vi "Varint Decoder uint64.vi"(7 "Optional":bool, 8 "error in (no error)":errorcluster, 9 "Array":u8[](array[numeric]) format="%02x", 10 "Key":i32=-1) -> (0 "error out":errorcluster, 1 "array w/ subset deleted":u8[](array[numeric]), 2 "Read Key":i32, 3 "Varint":u64)   [LabVIEW 2017]
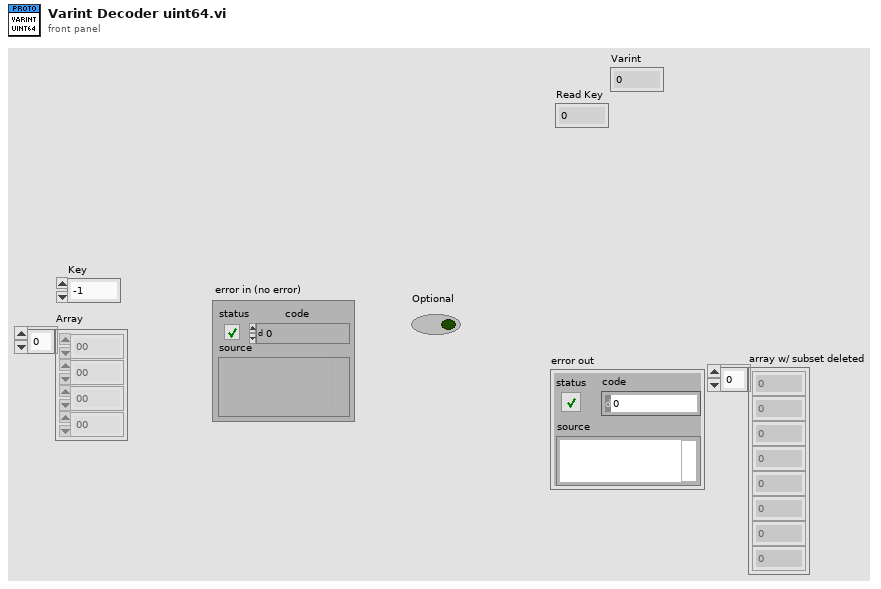
[diagram p1: front panel]
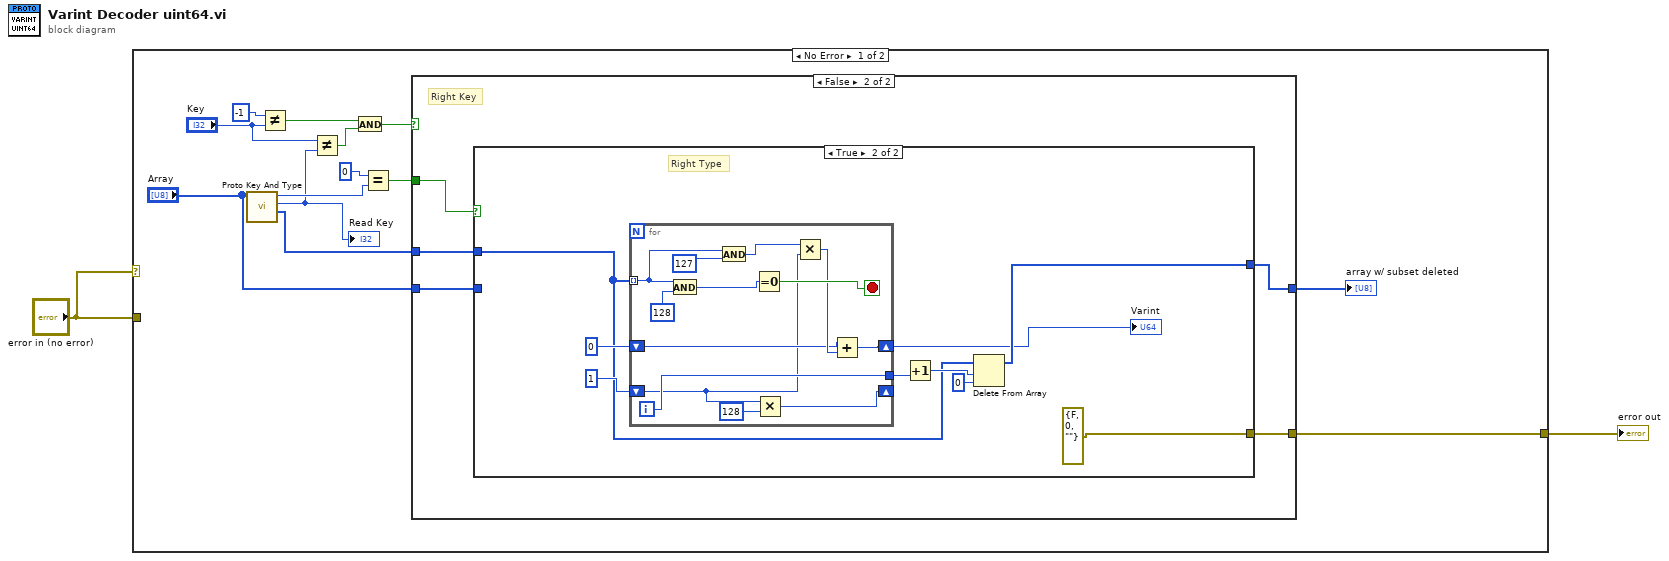
[diagram p0: block diagram]
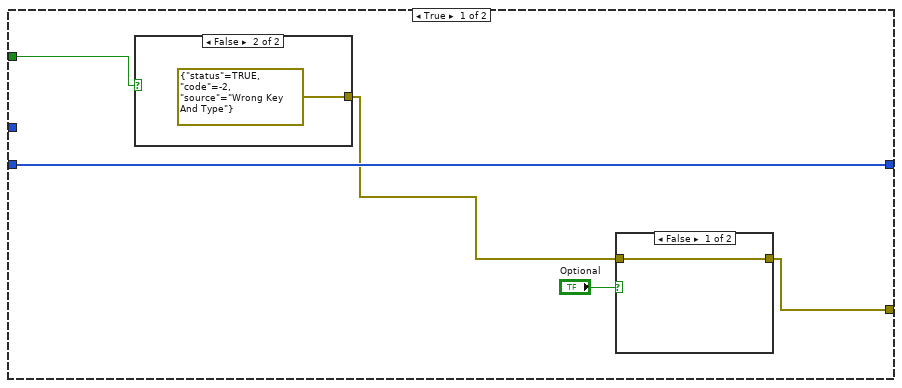
[diagram p2: hidden frame]
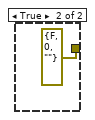
[diagram p3: hidden frame]
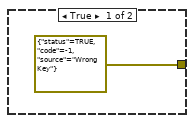
[diagram p4: hidden frame]
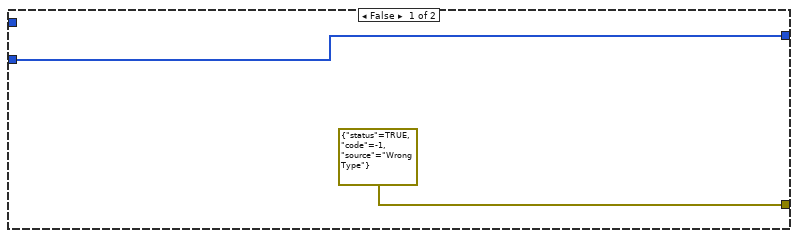
[diagram p5: hidden frame]
diagram:
  n1 = case shown="No Error" "error in (no error)" {
    tunnel: "error in (no error)" -> [_ w54]
    tunnel: [w3 w54] -> w1
    frame No Error {
      n2 = call "Proto Key And Type.vi"("Array"="Array") -> ("array w/ subset deleted"=w15:u8[], "Key"=w4:i32, "Type"=w7:i32)  [unwired: 8 in]
      "Read Key" <- w4
      n3 = Not Equal?(x=-1, y="Key") -> (x != y?=w12:bool)
      n4 = Not Equal?(x="Key", y=w4) -> (x != y?=w10:bool)
      n5 = And(x=w12, y=w10) -> (x .and. y?=w9:bool)
      n6 = Equal?(x=0, y=w7) -> (x = y?=w6:bool)
      n7 = case shown="False" w9 {
        tunnel: w15 -> [_ w29]
        tunnel: "Array" -> [w19 w28]
        tunnel: w6 -> [w20 w27]
        tunnel: [w17 w26] -> w3
        tunnel: [w19 w25] -> w5
        frame True {
          n8 = case shown="False" w20 {
            tunnel: [errorcluster {"status"=TRUE, "code"=-1, "source"="Wrong Key"} ("error in (no error)") errorcluster {"status"=TRUE, "code"=-2, "source"="Wrong Key And Type"} ("error in (no error)")] -> w16
            frame True {
            }
            frame False {
            }
          }
          n9 = case shown="False" "Optional" {
            tunnel: [w21 errorcluster {"status"=FALSE, "code"=0, "source"=""} ("error in (no error)")] -> w17
            tunnel: w16 -> [w21 _]
            frame False {
            }
            frame True {
            }
          }
        }
        frame False {
          # "Right Key"
          n10 = case shown="True" w27 {
            tunnel: [errorcluster {"status"=TRUE, "code"=-1, "source"="Wrong Type"} ("error in (no error)") errorcluster {"status"=FALSE, "code"=0, "source"=""} ("error in (no error)")] -> w26
            tunnel: w29 -> [_ w34]
            tunnel: [w30 w33] -> w25
            tunnel: w28 -> [w30 _]
            frame False {
            }
            frame True {
              # "Right Type"
              n11 = for {
                tunnel: w34 -> [w49] mode=indexing
                tunnel: [w50] -> w38
                shift-right: [w44] -> w32
                shift-left: u64 0 -> [w45]
                shift-right: [w42] -> _
                shift-left: u64 1 -> [w43]
                i -> [w50]
                stop <- w51 stop-if-true
                n12 = And(x=w49, y=u8 128 ("x")) -> (x .and. y?=w52:u8)
                n13 = And(x=w49, y=u8 127) -> (x .and. y?=w47:u8)
                n14 = Equal To 0?(x=w52) -> (x = 0?=w51:bool)
                n15 = Multiply(x=w43, y=u64 128) -> (x*y=w42:u64)
                n16 = Multiply(x=w47, y=w43) -> (x*y=w46:u64)
                n17 = Add(x=w45, y=w46) -> (x+y=w44:u64)
              }
              "Varint" <- w32
              n18 = Increment(x=w38) -> (x+1=w37:i32)
              n19 = Delete From Array(array=w34, length=w37, index=0) -> (array with subset deleted=w33:u8[])  [unwired: 1 out]
            }
          }
        }
      }
      "array w/ subset deleted" <- w5
    }
    frame Error {
    }
  }
  "error out" <- w1
